vi "글로벌 1.vi"() -> ()   [LabVIEW 2019]
panel:
  in  "문자열":string
  in  "불리언":bool
  in  "다이얼":dbl(knob) scale=0.0..10.0
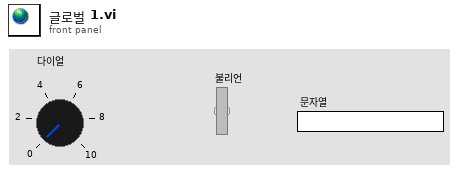
[diagram p1: front panel]
diagram:
